vi "Year2018_Q3.vi"() -> ()   [LabVIEW 2015]
panel:
  out "Sum of \nOdd numbers":dbl
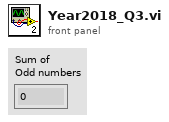
[diagram p1: front panel]
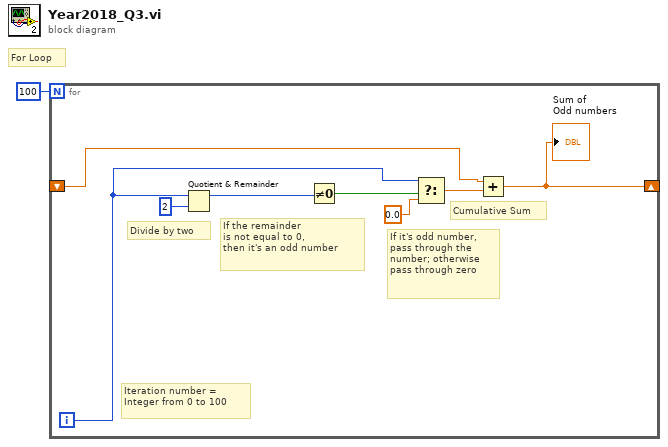
[diagram p0: block diagram]
diagram:
  # "For Loop"
  n1 = for {
    N: 100 -> [_]
    shift-right: [w2] -> _
    shift-left: _ -> [w3]
    i -> [w5]
    # "Cumulative Sum"
    # "If it's odd number,\npass through the \nnumber; otherwise\npass through zero"
    # "Divide by two"
    # "If the remainder\nis not equal to 0,\nthen it's an odd number"
    # "Iteration number = \nInteger from 0 to 100"
    n2 = Quotient & Remainder(x=w5, y=2) -> (x-y*floor(x/y)=w8:i32)  [unwired: 1 out]
    n3 = Not Equal To 0?(x=w8) -> (x != 0?=w7:bool)
    n4 = Select(t=w5, s=w7, f=0.0) -> (s? t:f=w4:dbl)
    n5 = Add(x=w3, y=w4) -> (x+y=w2:dbl)
    "Sum of \nOdd numbers" <- w2
  }
